vi "pm_load_node_sub.vi"(9 "offset":u32, 11 "Buffer":string) -> (0 "Next offset":u32, 1 "dataptr":u32, 3 "nchildren":u32, 8 "size":u32)   [LabVIEW 2017, in "HEKAdat.lvclass"]
uses:
  HEKAdat.lvclass
panel:
  in  "lvl_sizes":u32[](array[numeric])
  in  "nlevels":u32
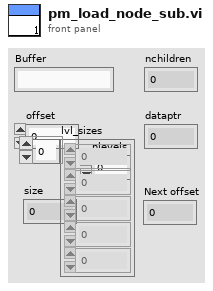
[diagram p1: front panel]
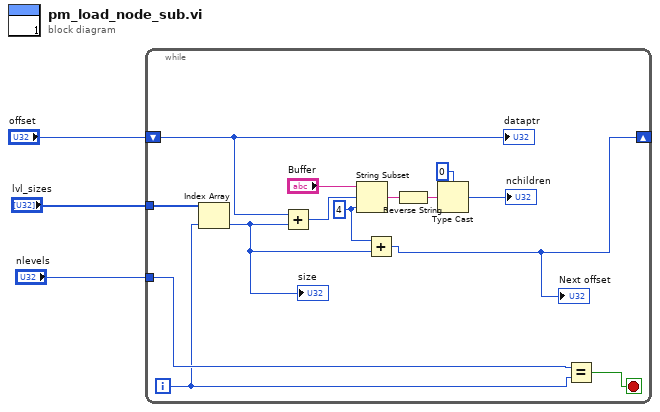
[diagram p0: block diagram]
diagram:
  n1 = while {
    tunnel: "nlevels" -> [w10]
    tunnel: "lvl_sizes" -> [w8]
    shift-right: [w4] -> _
    shift-left: "offset" -> [w5]
    i -> [w7]
    stop <- w9 stop-if-true
    w11 = u32 4 ("length (rest)")
    n2 = Index Array(array=w8, index=w7) -> (element=w6:u32)
    "size" <- w6
    n3 = Add(x=w5, y=w6) -> (x+y=w12:u32)
    n4 = String Subset(string="Buffer", offset (0)=w12, length (rest)=w11) -> (substring=w14:string)
    n5 = Add(x=w11, y=w6) -> (x+y=w4:u32)
    "Next offset" <- w4
    n6 = Reverse String(1:w14) -> (0:w15:string)
    n7 = Type Cast(type=u32 0, x=w15) -> (*(type *) &x=→"nchildren":u32)
    n8 = Equal?(x=w10, y=w7) -> (x = y?=w9:bool)
    "dataptr" <- w5
  }
